vi "QPSK (SubVI).vi"(11 "output bit stream":i8[](array[numeric])) -> (3 "Array":cdb[](array[numeric]))   [LabVIEW 2018]
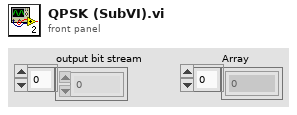
[diagram p1: front panel]
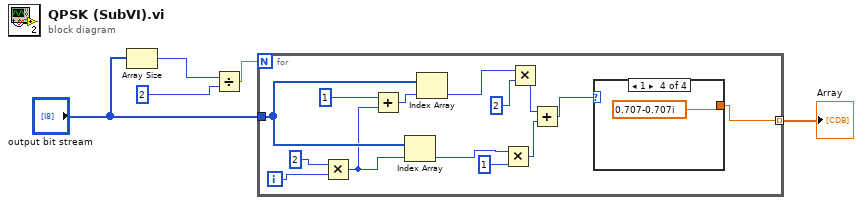
[diagram p0: block diagram]
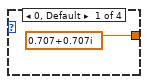
[diagram p2: hidden frame]
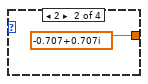
[diagram p3: hidden frame]
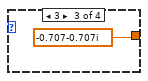
[diagram p4: hidden frame]
diagram:
  n1 = Array Size(array="output bit stream") -> (size(s)=w2:i32)
  n2 = Divide(x=w2, y=2) -> (x/y=w4:dbl)
  n3 = for {
    N: w4 -> [_]
    tunnel: "output bit stream" -> [w19]
    tunnel: [w7] -> w5 mode=indexing
    i -> [w14]
    n4 = Multiply(x=2, y=w14) -> (x*y=w16:i32)
    n5 = Add(x=1, y=w16) -> (x+y=w18:i32)
    n6 = Index Array(array=w19, index=w16) -> (element=w10:i8)
    n7 = Index Array(array=w19, index=w18) -> (element=w12:i8)
    n8 = Multiply(x=w10, y=1) -> (x*y=w8:i32)
    n9 = Multiply(x=w12, y=2) -> (x*y=w9:i32)
    n10 = Add(x=w9, y=w8) -> (x+y=w6:i32)
    n11 = case shown="1" w6 {
      tunnel: [cdb 0.707+0.707i cdb -0.707+0.707i cdb -0.707-0.707i cdb 0.707-0.707i] -> w7
      frame 0, Default {
      }
      frame 2 {
      }
      frame 3 {
      }
      frame 1 {
      }
    }
  }
  "Array" <- w5
